vi "PathPlanner_ModuleConfig_New.vi"(4 "Gearing":i32=1, 6 "NumMotors":i32, 7 "wheelRadiusMeters":dbl, 8 "driveCurrentLimit":dbl, 9 "driveMotor":T1 {"Jr_KgM2" format="%13.5p"; "L_H" format="%13.5p"; "Kt_NMPerAmp" format="%13.5p"; "KvINV_RadPerSecPerVolt" format="%13.5p"; "R_Ohms" format="%13.5p"; "FreeSpeed_RadPerSec" format="%13.5p"; "FreeCurrent_Amps" format="%13.5p"; "StallCurrent_Amps" format="%13.5p"; "StallTorque_NM" format="%13.5p"; "nominalVoltage_Volts" format="%13.5p"}, 10 "wheelCOF":dbl, 11 "maxDriveVelocityMPS":dbl) -> (3 "ModuleConfig":T2 {"driveMotor"."Jr_KgM2" format="%13.5p"; "driveMotor"."L_H" format="%13.5p"; "driveMotor"."Kt_NMPerAmp" format="%13.5p"; "driveMotor"."KvINV_RadPerSecPerVolt" format="%13.5p"; "driveMotor"."R_Ohms" format="%13.5p"; "driveMotor"."FreeSpeed_RadPerSec" format="%13.5p"; "driveMotor"."FreeCurrent_Amps" format="%13.5p"; "driveMotor"."StallCurrent_Amps" format="%13.5p"; "driveMotor"."StallTorque_NM" format="%13.5p"; "driveMotor"."nominalVoltage_Volts" format="%13.5p"})   [LabVIEW 2019, in "PathPlanner24.lvlib"]
doc: "Create a trajectory state\n\nInputs:\n -- timeSeconds - double - The time at this state in seconds ( default = 0; )\n -- velocityMps - double - The velocity at this state in m/s ( default = 0 )\n -- accelerationMpsSq - double - The acceleration at this state in m/s^2 ( default = 0 )\n -- headingAngularVelocityRps - double - The time at this state in seconds ( default = 0 )\n -- positionMeters - translation2d - The position at this state in meters ( default = 0,0 )\n -- heading - rotation2d - The heading (direction of travel) at this state ( default = 0 )\n -- targetHolonomicRotation - rotation2d - The target holonomic rotation at this state ( default = 0 )\n -- curvatureRadPerMeter - double - The curvature at this state in rad/m ( default = 0 )\n -- constraints -- cluster -- constraints to apply at this state (default - none )\n - WaypointRelPos - double - The waypoint relative pos for this state.\n\n\nOutputs\n - PathPlannerTrajectoryState -- cluster -- Newly created state"
uses:
  PathPlanner24.lvlib
  TypeDef/PathPlannerModuleConfig.ctl
  <vilib>/Rock Robotics/WPI/ThirdParty/JAS_Junk/TrajLib/TypeDef/DCMOTOR.CTL
  <vilib>/Rock Robotics/WPI/ThirdParty/JAS_Junk/TrajLib/Trajectory_Library.lvlib
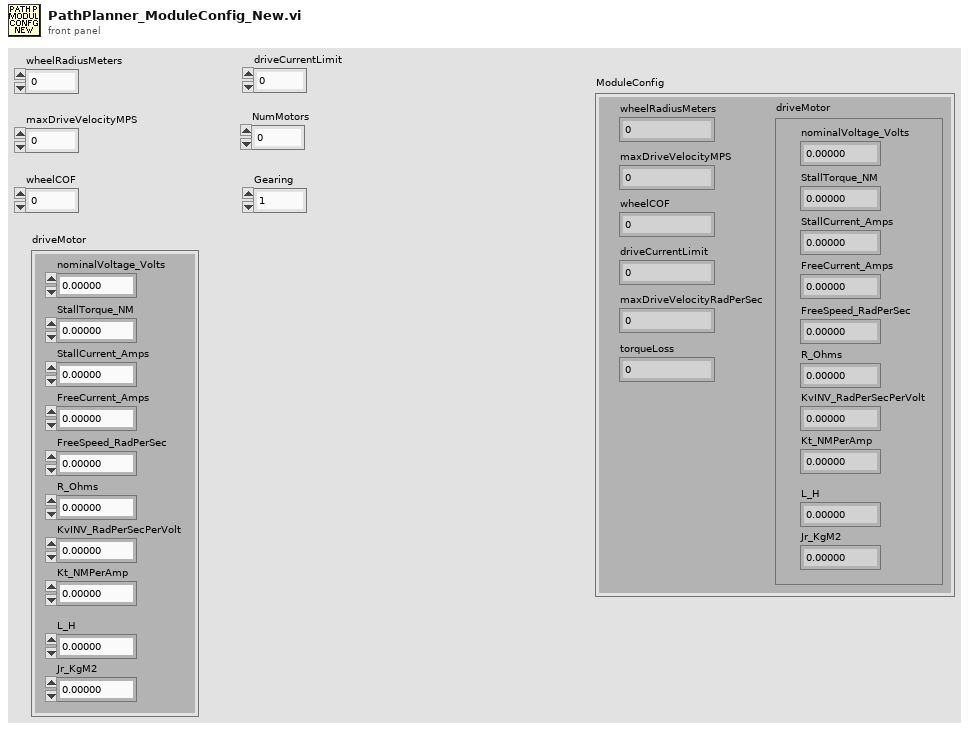
[diagram p1: front panel]
types:
  T1 = typedef "Trajectory_Library.lvlib/DCMOTOR.CTL" = cluster{"nominalVoltage_Volts":dbl, "StallTorque_NM":dbl, "StallCurrent_Amps":dbl, "FreeCurrent_Amps":dbl, "FreeSpeed_RadPerSec":dbl, "R_Ohms":dbl, "KvINV_RadPerSecPerVolt":dbl, "Kt_NMPerAmp":dbl, "L_H":dbl, "Jr_KgM2":dbl}
  T2 = typedef "PathPlanner24.lvlib/PathPlannerModuleConfig.ctl" = cluster{"wheelRadiusMeters":dbl, "maxDriveVelocityMPS":dbl, "wheelCOF":dbl, "driveCurrentLimit":dbl, "maxDriveVelocityRadPerSec":dbl, "torqueLoss":dbl, "driveMotor":T1}
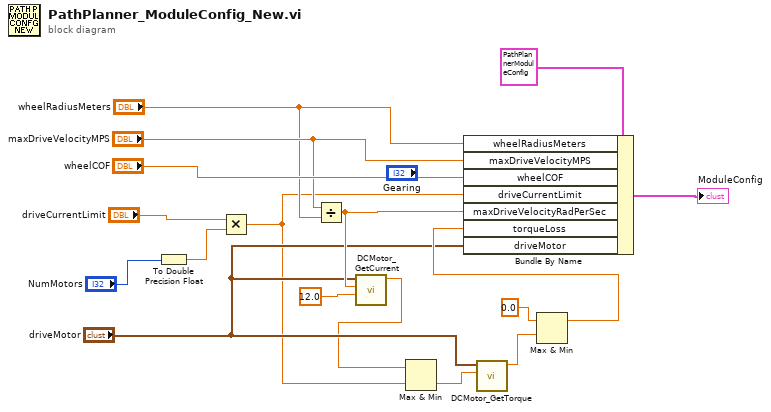
[diagram p0: block diagram]
diagram:
  n1 = To Double Precision Float(number="NumMotors") -> (double precision float=w13:dbl)
  n2 = Multiply(x="driveCurrentLimit", y=w13) -> (x*y=w2:dbl)
  n3 = Divide(x="maxDriveVelocityMPS", y="wheelRadiusMeters") -> (x/y=w9:dbl)
  n4 = call <vilib>:"DCMotor_GetCurrent.vi"("VoltageInput_Volts"=12.0, "Speed_RadPerSec"=w9, "DCMOTOR"="driveMotor") -> ("Current_Amps"=w1:dbl)  [unwired: 8 in]
  n5 = Max & Min(x=w1, y=w2) -> (min(x,y)=w3:dbl)  [unwired: 1 out]
  n6 = call <vilib>:"DCMotor_GetTorque.vi"("Current_Amps"=w3, "DCMOTOR"="driveMotor") -> ("Torque_KtNM"=w5:dbl)  [unwired: 9 in]
  n7 = Max & Min(x=0.0, y=w5) -> (max(x,y)=w7:dbl)  [unwired: 1 out]
  n8 = Bundle By Name(cluster=T2 {"wheelRadiusMeters"=0.0, "maxDriveVelocityMPS"=0.0, "wheelCOF"=0.0, "driveCurrentLimit"=0.0, "maxDriveVelocityRadPerSec"=0.0, "torqueLoss"=0.0, "driveMotor"={"nominalVoltage_Volts"=0.0, "StallTorque_NM"=0.0, "StallCurrent_Amps"=0.0, "FreeCurrent_Amps"=0.0, "FreeSpeed_RadPerSec"=0.0, "R_Ohms"=0.0, "KvINV_RadPerSecPerVolt"=0.0, "Kt_NMPerAmp"=0.0, "L_H"=0.0, "Jr_KgM2"=0.0}} ("PathPlannerState"), "wheelRadiusMeters"="wheelRadiusMeters", "maxDriveVelocityMPS"="maxDriveVelocityMPS", "wheelCOF"="wheelCOF", "driveCurrentLimit"=w2, "maxDriveVelocityRadPerSec"=w9, "torqueLoss"=w7, "driveMotor"="driveMotor") -> (→"ModuleConfig":T2)
